vi "一维数组冒泡排序.vi"(1 "输入":dbl[](array[numeric])) -> (0 "输出":dbl[](array[numeric]))   [LabVIEW 2014]
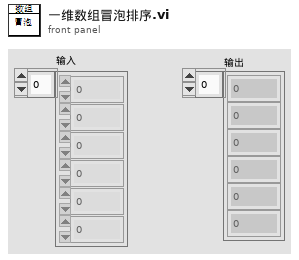
[diagram p1: front panel]
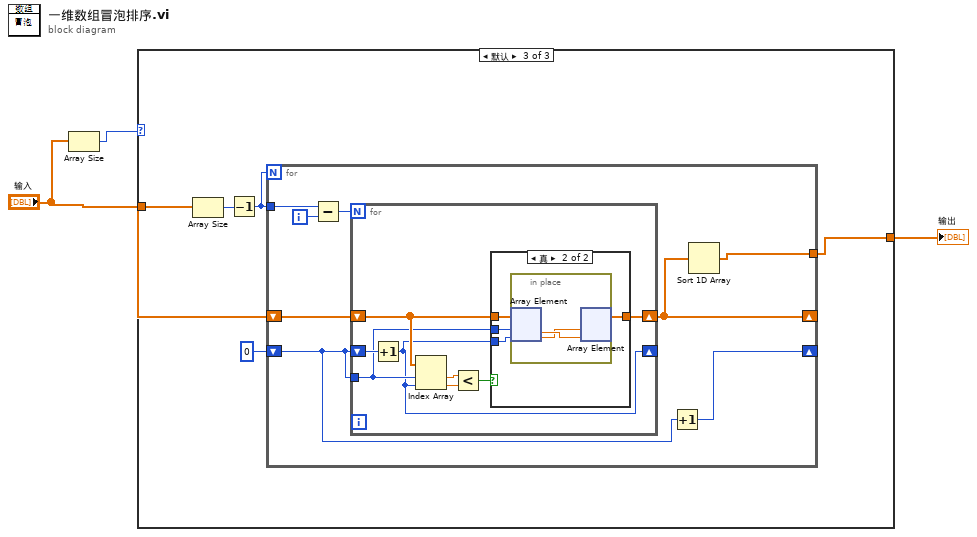
[diagram p0: block diagram]
diagram:
  n1 = Array Size(array="输入") -> (size(s)=w2:i32)
  n2 = case shown="默认" w2 {
    tunnel: "输入" -> [w4 w5 w9]
    tunnel: [w4 w5 w6] -> w1
    frame 0 {
    }
    frame 1 {
    }
    frame Default {
      n3 = Array Size(array=w9) -> (size(s)=w10:i32)
      n4 = Decrement(x=w10) -> (x-1=w8:i32)
      n5 = for {
        N: w8 -> [_]
        tunnel: w8 -> [w17]
        shift-right: [w12] -> _
        shift-left: w9 -> [w18]
        shift-right: [w14] -> _
        shift-left: 0 -> [w13]
        tunnel: [w11] -> w6
        i -> [w16]
        n6 = Subtract(x=w17, y=w16) -> (x-y=w15:i32)
        n7 = for {
          N: w15 -> [_]
          shift-right: [w25] -> w12
          shift-left: w18 -> [w24]
          shift-right: [w19] -> _
          shift-left: w13 -> [w21]
          tunnel: w13 -> [w20]
          n8 = Increment(x=w21) -> (x+1=w19:i32)
          n9 = Index Array(array=w24, index #1=w20, index #2=w19) -> (element #1=w23:dbl, element #2=w22:dbl)
          n10 = Less?(x=w23, y=w22) -> (x < y?=w26:bool)
          n11 = case shown="真" w26 {
            tunnel: w24 -> [w27 w31]
            tunnel: [w27 w30] -> w25
            tunnel: w20 -> [_ w29]
            tunnel: w19 -> [_ w28]
            frame False {
            }
            frame True {
              n12 = in-place {
                n13 = in-place-array #1(w31, w29, w28) -> (w33:dbl, w32:dbl)
                n14 = in-place-array #1(w32, w33) -> (w30:dbl[])  [unwired: 2 out]
              }
            }
          }
        }
        n15 = Increment(x=w13) -> (x+1=w14:i32)
        n16 = Sort 1D Array(array=w12) -> (sorted array=w11:dbl[])
      }
    }
  }
  "输出" <- w1
